vi "Gunsim Initial Position.vi"(1 "Parameters":T3, 2 "Robot Constants":T1={"Distance from Pivot Point to Drive Mount(in)"=2.0, "Distance from Pivot Point to Arm Mount(in)"=2.0, "Distance from Pivot Point to Launcher(in)"=2.0, "Distance from Pivot Point to Camera(in)"=2.0, "WheelEncoder Ticks/Revolution"=2.0, "Wheel Radius"=2.0, "Triangle Angle(degrees)"=2.0, "Minimum LA Distance(inches)"=2.0, "LA Distance/Tick(inches)"=2.0}, 3 "cluster in":T2={"Drag"=0.0, "gravity(in/s^2)"=-386.09, "Minimum Goal Height(in)"=85.0, "Maximum Goal Height(in)"=109.0, "xspeed"=0.0, "yspeed"=0.0, "xpos"=0.0, "ypos"=0.0, "Frametime"=0.0, "Graph Array 0"=[], "Graph Array 1"=[], "Output Array"=[]}) -> (0 "cluster out":T2)   [LabVIEW 2015]
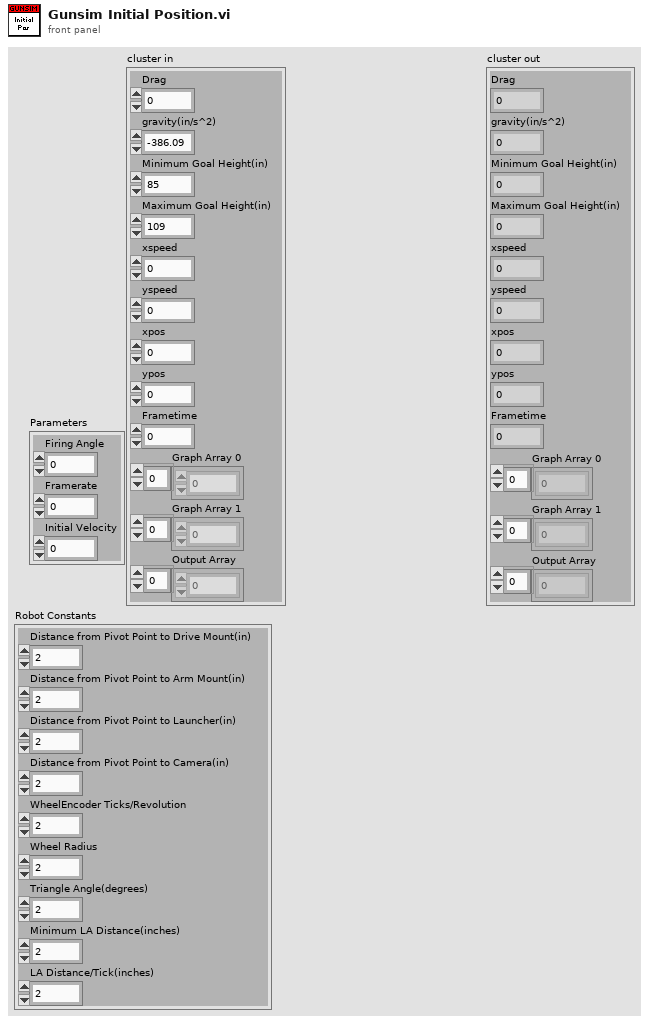
[diagram p1: front panel]
types:
  T1 = cluster{"Distance from Pivot Point to Drive Mount(in)":dbl, "Distance from Pivot Point to Arm Mount(in)":dbl, "Distance from Pivot Point to Launcher(in)":dbl, "Distance from Pivot Point to Camera(in)":dbl, "WheelEncoder Ticks/Revolution":dbl, "Wheel Radius":dbl, "Triangle Angle(degrees)":dbl, "Minimum LA Distance(inches)":dbl, "LA Distance/Tick(inches)":dbl}
  T2 = cluster{"Drag":dbl, "gravity(in/s^2)":dbl, "Minimum Goal Height(in)":dbl, "Maximum Goal Height(in)":dbl, "xspeed":dbl, "yspeed":dbl, "xpos":dbl, "ypos":dbl, "Frametime":dbl, "Graph Array 0":dbl[], "Graph Array 1":dbl[], "Output Array":dbl[]}
  T3 = cluster{"Firing Angle":dbl, "Framerate":dbl, "Initial Velocity":dbl}
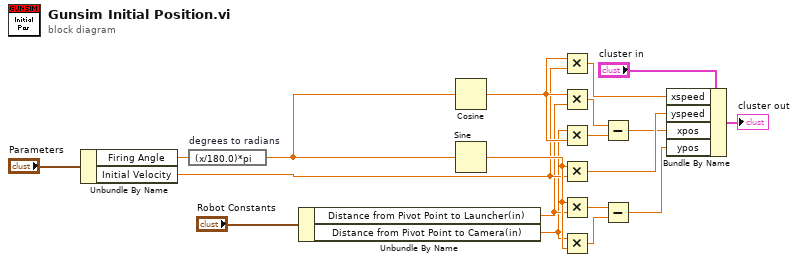
[diagram p0: block diagram]
diagram:
  n1 = Unbundle By Name("Parameters") -> ("Firing Angle"=w17:dbl, "Initial Velocity"=w4:dbl)
  n2 = expression code="(x/180.0)*pi" "degrees to radians"(w17) -> (w14:dbl)
  n3 = Unbundle By Name("Robot Constants") -> ("Distance from Pivot Point to Launcher(in)"=w3:dbl, "Distance from Pivot Point to Camera(in)"=w2:dbl)
  n4 = Cosine(x=w14) -> (cos(x)=w11:dbl)
  n5 = Sine(x=w14) -> (sin(x)=w9:dbl)
  n6 = Multiply(x=w11, y=w4) -> (x*y=w19:dbl)
  n7 = Multiply(x=w11, y=w3) -> (x*y=w12:dbl)
  n8 = Multiply(x=w2, y=w11) -> (x*y=w10:dbl)
  n9 = Multiply(x=w9, y=w4) -> (x*y=w18:dbl)
  n10 = Multiply(x=w9, y=w3) -> (x*y=w13:dbl)
  n11 = Multiply(x=w2, y=w9) -> (x*y=w8:dbl)
  n12 = Subtract(x=w12, y=w10) -> (x-y=w6:dbl)
  n13 = Subtract(x=w13, y=w8) -> (x-y=w7:dbl)
  n14 = Bundle By Name(cluster="cluster in", "xspeed"=w19, "yspeed"=w18, "xpos"=w6, "ypos"=w7) -> (→"cluster out":T2)
